vi "Asynchronous VI launcher.vi"() -> ()   [LabVIEW 2021]
panel:
  out "reference out":refnum<vi>
  out "error out":errorcluster
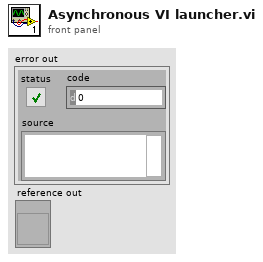
[diagram p1: front panel]
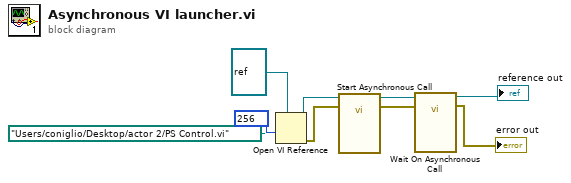
[diagram p0: block diagram]
diagram:
  n1 = Open VI Reference(type specifier VI Refnum (for type only)=refnum<vi> refnum, vi path=path "/Users/coniglio/Desktop/actor 2/PS Control.vi", options=256) -> (vi reference=w1:refnum<vi>, error out=w2:errorcluster)  [unwired: 3 in]
  n2 = call-by-ref "Start Asynchronous Call"(reference=w1, error in=w2) -> (reference out=w9:refnum<vi>, error out=w8:errorcluster)  [unwired: 12 in]
  n3 = call-by-ref "Wait On Asynchronous Call"(reference=w9, error in=w8) -> (reference out=→"reference out":refnum<vi>, error out=→"error out":errorcluster)  [unwired: 12 in]
